vi "Zedver_v3_CSVtoString_DEFI.vi"(6 "PROCE CSV":path, 7 "RAW Activ.":bool, 8 "HISTO CSV":path, 9 "RAW CSV":path, 10 "Process Activ.":bool, 11 "Histogram Activ.":bool) -> (0 "concatenated string":string, 1 "Process bytes":u16, 2 "Histogram bytes":u16, 3 "Raw bytes":u16)   [LabVIEW 2011]
uses:
  <vilib>/Utility/file.llb/Read From Spreadsheet File (DBL).vi
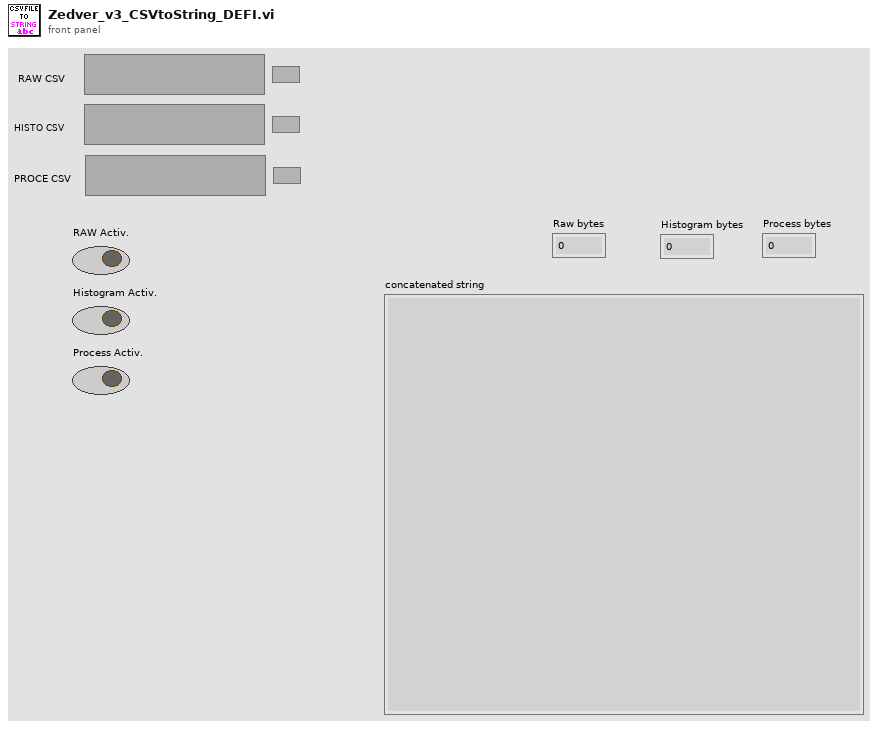
[diagram p1: front panel]
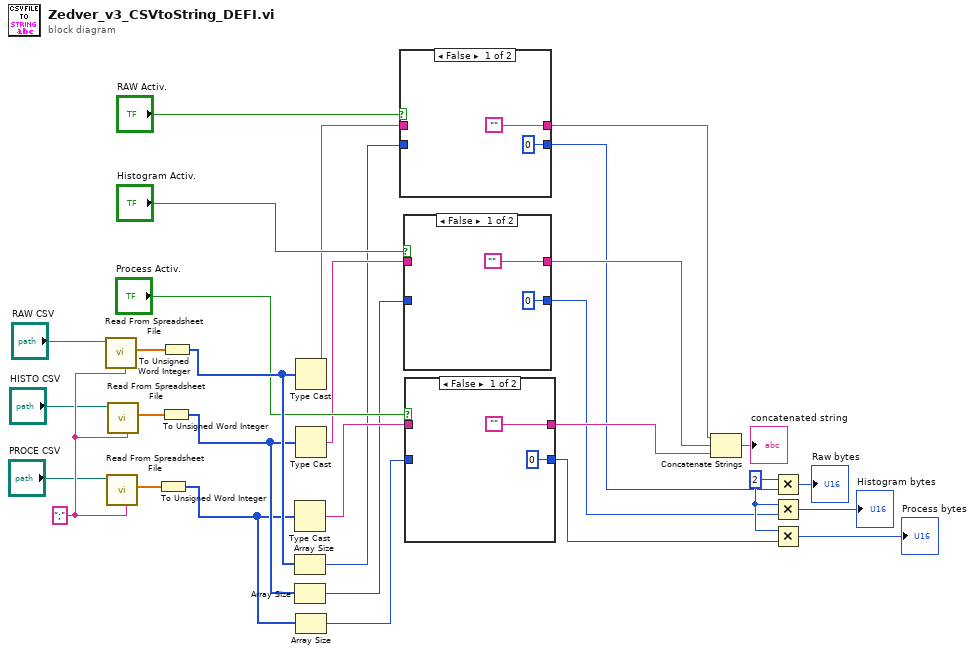
[diagram p0: block diagram]
diagram:
  w19 = 2 ("x")
  w30 = ";" ("delimiter (\\t)")
  n1 = call-poly <vilib>:"Read From Spreadsheet File.vi"("delimiter (\\t)"=w30, "file path (dialog if empty)"="RAW CSV") -> ("first row"=w26:dbl[])  [unwired: 5 in, 4 out]
  n2 = call-poly <vilib>:"Read From Spreadsheet File.vi"("delimiter (\\t)"=w30, "file path (dialog if empty)"="PROCE CSV") -> ("first row"=w24:dbl[])  [unwired: 5 in, 4 out]
  n3 = call-poly <vilib>:"Read From Spreadsheet File.vi"("delimiter (\\t)"=w30, "file path (dialog if empty)"="HISTO CSV") -> ("first row"=w25:dbl[])  [unwired: 5 in, 4 out]
  n4 = To Unsigned Word Integer(number=w24) -> (unsigned 16bit integer=w20:u16[])
  n5 = To Unsigned Word Integer(number=w25) -> (unsigned 16bit integer=w21:u16[])
  n6 = To Unsigned Word Integer(number=w26) -> (unsigned 16bit integer=w22:u16[])
  n7 = Type Cast(x=w20) -> (*(type *) &x=w10:string)  [unwired: 1 in]
  n8 = Array Size(array=w22) -> (size(s)=w4:i32)
  n9 = Array Size(array=w21) -> (size(s)=w5:i32)
  n10 = Type Cast(x=w22) -> (*(type *) &x=w12:string)  [unwired: 1 in]
  n11 = Type Cast(x=w21) -> (*(type *) &x=w11:string)  [unwired: 1 in]
  n12 = Array Size(array=w20) -> (size(s)=w6:i32)
  n13 = case shown="False" "RAW Activ." {
    tunnel: ["" w34] -> w9
    tunnel: w12 -> [_ w34]
    tunnel: w4 -> [_ w33]
    tunnel: [u16 0 w33] -> w1
    frame False {
    }
    frame True {
    }
  }
  n14 = case shown="False" "Histogram Activ." {
    tunnel: ["" w38] -> w7
    tunnel: w11 -> [_ w38]
    tunnel: w5 -> [_ w37]
    tunnel: [u16 0 w37] -> w2
    frame False {
    }
    frame True {
    }
  }
  n15 = case shown="False" "Process Activ." {
    tunnel: ["" w42] -> w8
    tunnel: w10 -> [_ w42]
    tunnel: w6 -> [_ w41]
    tunnel: [u16 0 w41] -> w3
    frame False {
    }
    frame True {
    }
  }
  n16 = Concatenate Strings(w9, w7, w8) -> (→"concatenated string":string)
  n17 = Multiply(x=w19, y=w1) -> (x*y=→"Raw bytes":i32)
  n18 = Multiply(x=w19, y=w2) -> (x*y=→"Histogram bytes":i32)
  n19 = Multiply(x=w19, y=w3) -> (x*y=→"Process bytes":i32)
